vi "EditOptions.vi"(8 "error in":errorcluster, 11 "channel in":refnum<class "StepNode.lvclass">) -> (0 "error out":errorcluster, 1 "edit options":T1, 2 "subnodes class":T2, 3 "channel out":refnum<class "StepNode.lvclass">)   [LabVIEW 2015, in "StepNode.lvclass"]
doc: "This VI Contains the options for the Menu that will be displayed when doing right click on an item\nThe subnodes class configures which nodes can be added to this nodes\nAnd the edit options determine which options are available for the node.\n\nThis configuration is stored in this VI in case some dynamic configuration is required for the menu options or subnodes.\n\nAll VIs must overide this methodCopyright 2017 National Instruments Corporation\n\nLicensed under the Apache License, Version 2.0 (the \"License\"); you may not use this file except in compliance with the License. You may obtain a copy of the License at http://www.apache.org/licenses/LICENSE-2.0\nUnless required by applicable law or agreed to in writing, software distributed under the License is distributed on an \"AS IS\" BASIS, WITHOUT WARRANTIES OR CONDITIONS OF ANY KIND, either express or implied. See the License for the specific language governing permissions and limitations under the License."
uses:
  StepNode.lvclass
  <vilib>/NI/Configuration Framework/Node/SubNodeCluster.ctl
  <vilib>/NI/Configuration Framework/Node/NodeMenuOptions.ctl
  <vilib>/NI/Configuration Framework/Node/NISE_CEF_Node.lvclass
  Configuration Tool.lvlib
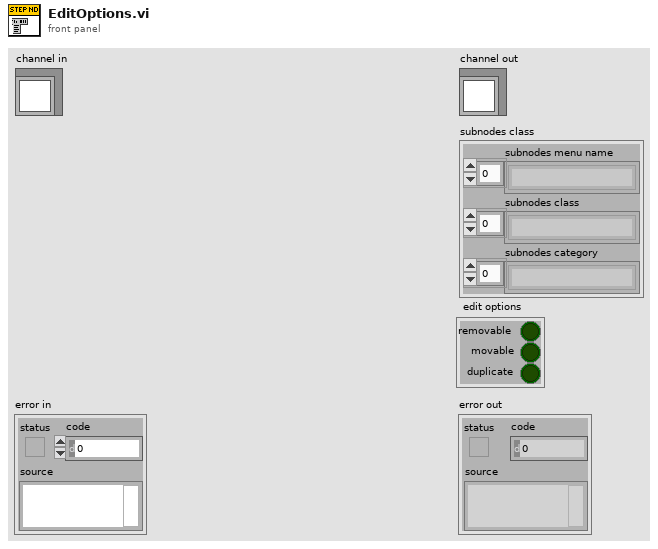
[diagram p1: front panel]
types:
  T1 = typedef "NISE_CEF_Node.lvclass/NodeMenuOptions.ctl" = cluster{"removable":bool, "movable":bool, "duplicate":bool}
  T2 = typedef "NISE_CEF_Node.lvclass/SubNodeCluster.ctl" = cluster{"subnodes menu name":string[], "subnodes class":string[], "subnodes category":string[]}
  T3 = typedef "Configuration Tool.lvlib/StepClassLibrary.ctl" = cluster{"Step Types":string[], "Step Config Classes":refnum<class "Step Config.lvclass">[]}
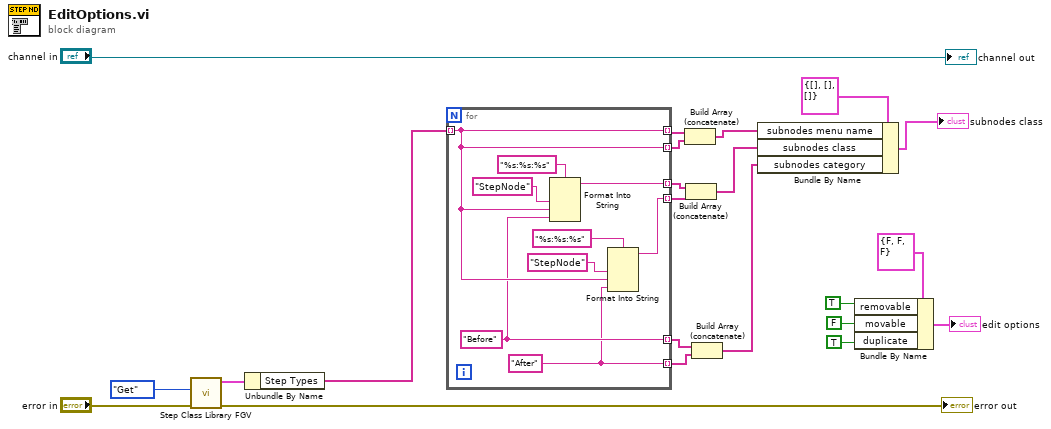
[diagram p0: block diagram]
diagram:
  n1 = call "Step Class Library FGV.vi"("error in (no error)"="error in", "Action"=enum16{"Set", "Get"}."Get") -> ("error out"=→"error out":errorcluster, "Step Type Class Library out"=w11:T3)  [unwired: 8 in]
  n2 = Unbundle By Name(w11) -> ("Step Types"=w10:string[])
  n3 = for {
    tunnel: w10 -> [w26] mode=indexing
    tunnel: [w25] -> w15 mode=indexing
    tunnel: [w31] -> w14 mode=indexing
    tunnel: [w26] -> w18 mode=indexing
    tunnel: [w26] -> w17 mode=indexing
    tunnel: [w24] -> w7 mode=indexing
    tunnel: [w23] -> w6 mode=indexing
    w23 = "After" ("Class")
    w24 = "Before" ("Class")
    n4 = Format Into String(format string="%s:%s:%s", "StepNode", w26, w24) -> (resulting string=w31:string)  [unwired: 2 in, 1 out]
    n5 = Format Into String(format string="%s:%s:%s", "StepNode", w26, w23) -> (resulting string=w25:string)  [unwired: 2 in, 1 out]
  }
  n6 = Build Array (concatenate)(w18, w17) -> (w16:string[])
  n7 = Build Array (concatenate)(w14, w15) -> (w13:string[])
  n8 = Build Array (concatenate)(w7, w6) -> (w5:string[])
  n9 = Bundle By Name(cluster=T2 {"subnodes menu name"=[], "subnodes class"=[], "subnodes category"=[]} ("subnodes class"), "subnodes menu name"=w16, "subnodes class"=w13, "subnodes category"=w5) -> (→"subnodes class":T2)
  n10 = Bundle By Name(cluster=T1 {"removable"=FALSE, "movable"=FALSE, "duplicate"=FALSE} ("edit options 2"), "removable"=TRUE ("movable"), "movable"=FALSE, "duplicate"=TRUE ("movable")) -> (→"edit options":T1)
  "channel out" <- "channel in"
